vi "Scale UI.vi"() -> ()   [LabVIEW 2011]
panel:
  out "error out":errorcluster
  in  "error in":errorcluster
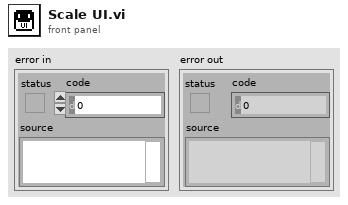
[diagram p1: front panel]
types:
  T1 = typedef "LVPointTypeDef.ctl" = cluster{"Horizontal":i16, "Vertical":i16}
  T2 = typedef "LVRectTypeDef.ctl" = cluster{"left":i16, "top":i16, "right":i16, "bottom":i16}
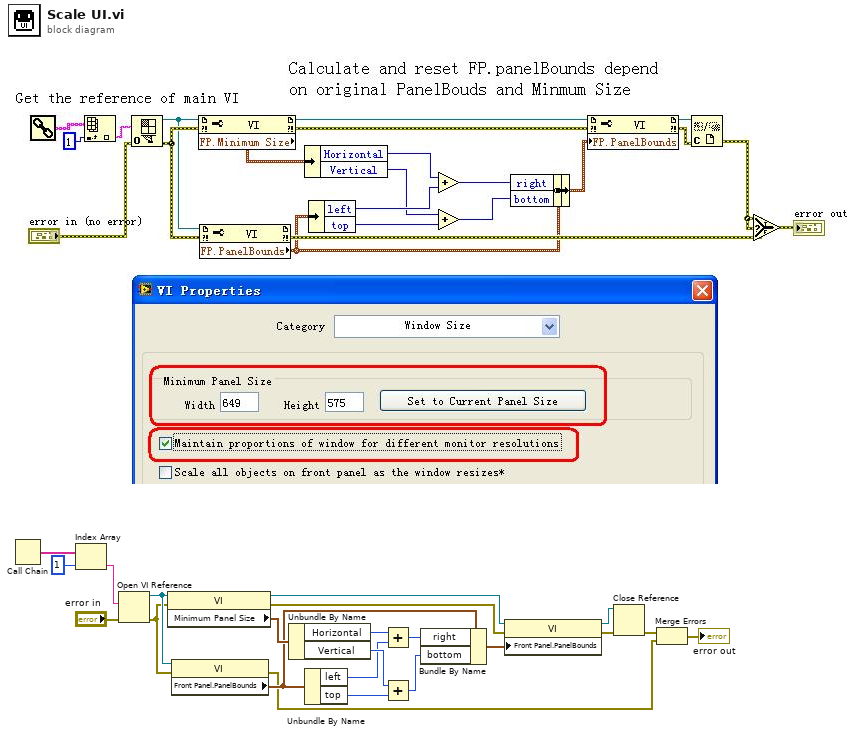
[diagram p0: block diagram]
diagram:
  n1 = Call Chain() -> (call chain=w22:string[])
  n2 = Index Array(array=w22, index=1) -> (element=w20:string)
  n3 = Open VI Reference(vi path=w20, error in (no error)="error in") -> (vi reference=w19:refnum<vi>, error out=w4:errorcluster)  [unwired: 4 in]
  n4 = property class="VI"(reference=w19, error in=w4) -> (reference out=w8:refnum<vi>, error out=w9:errorcluster, "Minimum Panel Size"=w18:T1)
  n5 = property class="VI"(reference=w19, error in=w4) -> (error out=w1:errorcluster, "Front Panel.PanelBounds"=w13:T2)  [unwired: 1 out]
  n6 = Unbundle By Name(w18) -> ("Horizontal"=w17:i16, "Vertical"=w16:i16)
  n7 = Unbundle By Name(w13) -> ("left"=w15:i16, "top"=w14:i16)
  n8 = Add(x=w17, y=w15) -> (x+y=w12:i16)
  n9 = Add(x=w16, y=w14) -> (x+y=w11:i16)
  n10 = Bundle By Name(cluster=w13, "right"=w12, "bottom"=w11) -> (w10:T2)
  n11 = property class="VI"(reference=w8, error in=w9, "Front Panel.PanelBounds"=w10) -> (reference out=w7:refnum<vi>, error out=w6:errorcluster)
  n12 = Close Reference(reference=w7, error in (no error)=w6) -> (error out=w2:errorcluster)
  n13 = Merge Errors(w2, w1) -> (→"error out":errorcluster)
